vi "Search Score Entry Array.vi"(8 "error in (no error)":errorcluster, 10 "Item Name":string, 11 "Array":string[][](array[string])) -> (0 "error out":errorcluster, 1 "Found?":bool, 2 "Value":string, 3 "Array Out":string[][](array[string]))   [LabVIEW 2013]
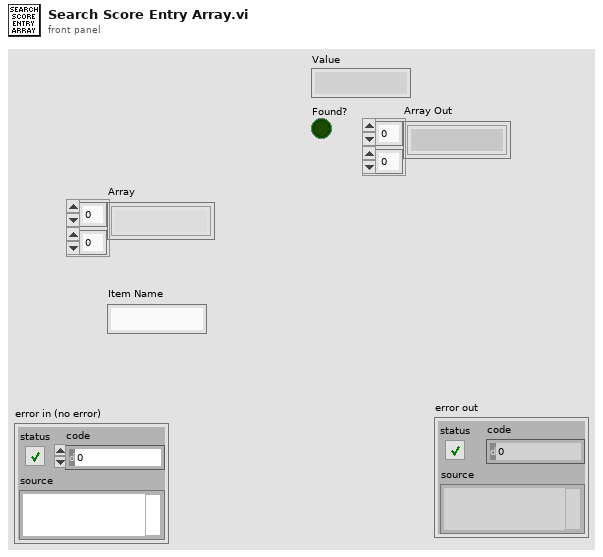
[diagram p1: front panel]
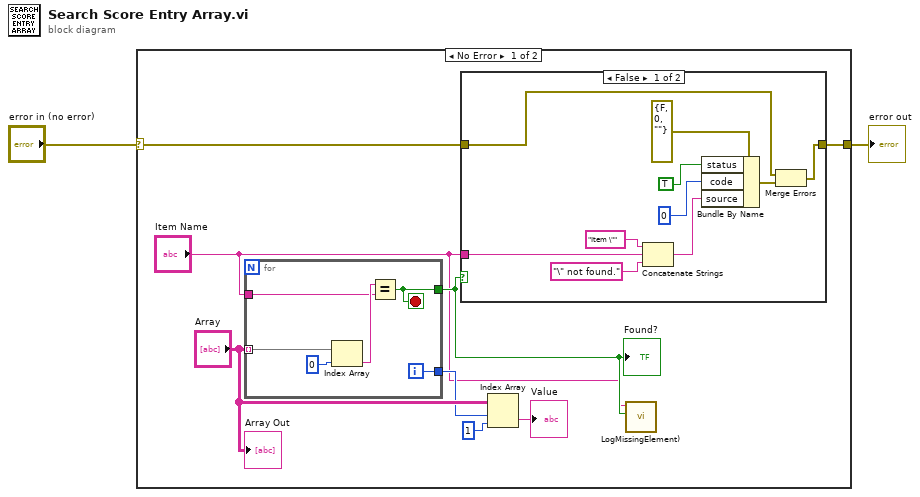
[diagram p0: block diagram]
diagram:
  n1 = case shown="No Error" "error in (no error)" {
    selector: "error in (no error)" -> [w6 w28]
    tunnel: [w5 w28] -> w1
    frame No Error {
      n2 = for {
        tunnel: "Array" -> [w27] mode=indexing
        tunnel: "Item Name" -> [w24]
        tunnel: [w23] -> w9
        tunnel: [w22] -> w4
        i -> [w23]
        stop <- w22 stop-if-true
        n3 = Index Array(array=w27, index=0) -> (element=w25:string)
        n4 = Equal?(x=w25, y=w24) -> (x = y?=w22:bool)
      }
      "Found?" <- w4
      n5 = case shown="False" w4 {
        tunnel: w6 -> [w20 w21]
        tunnel: [w19 w21] -> w5
        tunnel: "Item Name" -> [w13 _]
        frame False {
          n6 = Concatenate Strings("Item \"" ("string"), w13, "\" not found." ("string")) -> (w11:string)
          n7 = Bundle By Name(cluster=errorcluster {"status"=FALSE, "code"=0, "source"=""} ("error in"), "status"=TRUE, "code"=0, "source"=w11) -> (w17:errorcluster)
          n8 = Merge Errors(w20, w17) -> (w19:errorcluster)
        }
        frame True {
        }
      }
      n9 = Index Array(array="Array", index (row)=w9, index (col)=1 ("disabled index (col)")) -> (element=→"Value":string)
      n10 = call "LogMissingElement).vi"("Found?"=w4, "result string"="Item Name") -> ()  [unwired: 10 in]
      "Array Out" <- "Array"
    }
    frame Error {
    }
  }
  "error out" <- w1
